vi "Error Query.vi"(0 "VISA resource name":refnum<visa-resource-name>, 11 "error in (no error)":errorcluster {"code" format="%.0x"}) -> (4 "VISA resource name out":refnum<visa-resource-name>, 8 "Error":i32, 10 "Error Message":string, 15 "error out":errorcluster {"code" format="%.0x"})   [LabVIEW 2017, in "Agilent N6700 Series.lvlib"]
doc: "This VI reads an error code and a message from the instrument's error queue.\n\n<b>Note:</b>\n\nThis VI is called automatically by most driver VIs so it is not usually necessary to call this in an application."
uses:
  Agilent N6700 Series.lvlib
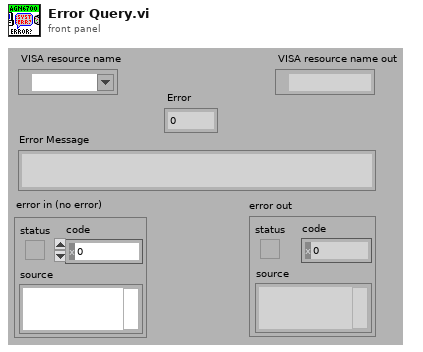
[diagram p1: front panel]
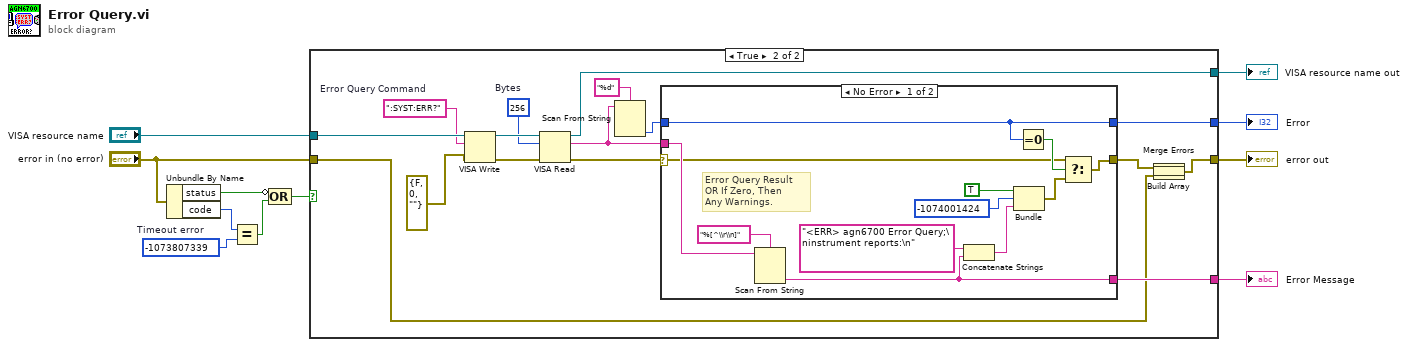
[diagram p0: block diagram]
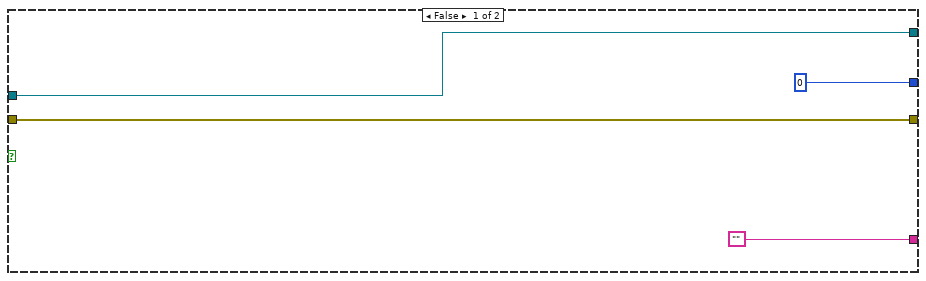
[diagram p2: hidden frame]
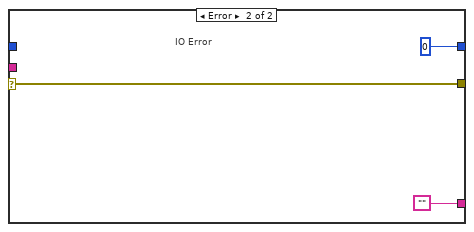
[diagram p3: hidden frame]
diagram:
  w4 = -1073807339  # Timeout error
  n1 = Unbundle By Name("error in (no error)") -> ("status"=w5:bool, "code"=w2:i32)
  n2 = Equal?(x=w2, y=w4) -> (x = y?=w3:bool)
  n3 = Compound Arithmetic op=OR(invert w5, w3) -> (w1:bool)
  n4 = case shown="True" w1 {
    tunnel: ["" ("Empty String Constant") w32] -> w11
    tunnel: [0 w31] -> w10
    tunnel: [w15 w30] -> w9
    tunnel: "VISA resource name" -> [w15 w29]
    tunnel: "error in (no error)" -> [w12 w22]
    tunnel: [w12 w21] -> w7
    frame False {
    }
    frame True {
      w27 = u32 256  # Bytes
      w25 = ":SYST:ERR?"  # Error Query Command
      n5 = VISA Write(VISA resource name=w29, write buffer=w25, error in (no error)=errorcluster {"status"=FALSE, "code"=0, "source"=""}) -> (VISA resource name out=w28:refnum<visa-resource-name>, error out=w26:errorcluster)  [unwired: 1 out]
      n6 = VISA Read(VISA resource name=w28, byte count=w27, error in (no error)=w26) -> (VISA resource name out=w30:refnum<visa-resource-name>, read buffer=w20:string, error out=w17:errorcluster)  [unwired: 1 out]
      n7 = Scan From String(format string="%d", input string=w20) -> (output 1=w18:i32)  [unwired: 3 in, 3 out]
      n8 = case shown="No Error" w17 {
        selector: w17 -> [w33 w45]
        tunnel: w20 -> [w35 _]
        tunnel: [w40 w45] -> w23
        tunnel: [w36 "" ("Empty String Constant")] -> w32
        tunnel: [w34 0] -> w31
        tunnel: w18 -> [w34 _]
        frame No Error {
          # "Error Query Result\nOR If Zero, Then\nAny Warnings."
          n9 = Scan From String(format string="%[^\\r\\n]", input string=w35) -> (output 1=w36:string)  [unwired: 3 in, 3 out]
          n10 = Concatenate Strings("<ERR> agn6700 Error Query;\ninstrument reports:\n" ("Source"), w36) -> (w42:string)
          n11 = Bundle("Status"=TRUE, "Code"=-1074001424, w42) -> (w41:cluster{"Status":bool, "Code":i32, string})  [unwired: 1 in]
          n12 = Equal To 0?(x=w34) -> (x = 0?=w38:bool)
          n13 = Select(t=w33, s=w38, f=w41) -> (s? t:f=w40:errorcluster)
        }
        frame Error {
          # "IO Error"
        }
      }
      n14 = Build Array(w23, w22) -> (w16:errorcluster[])
      n15 = Merge Errors(w16) -> (w21:errorcluster)
    }
  }
  "Error Message" <- w11
  "Error" <- w10
  "VISA resource name out" <- w9
  "error out" <- w7
